vi "close references.vi"(8 "error in":errorcluster, 11 "initialized references":T1[](array[typedef])) -> (0 "error out":errorcluster)   [LabVIEW 2013]
uses:
  Controls/initialized references.ctl
  Controls/interface VI type.ctl
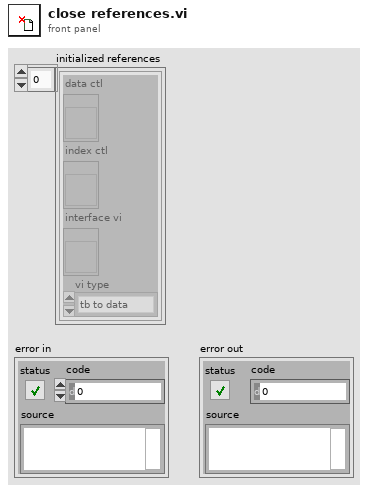
[diagram p1: front panel]
types:
  T1 = typedef "initialized references.ctl" = cluster{"data ctl":refnum<vi>, "index ctl":refnum<vi>, "interface vi":refnum<vi>, "vi type":T2}
  T2 = typedef "interface VI type.ctl" = enum16{"tb to data", "data to tb"}
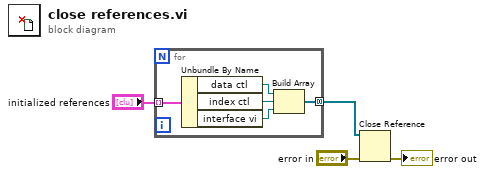
[diagram p0: block diagram]
diagram:
  n1 = for {
    tunnel: "initialized references" -> [w9] mode=indexing
    tunnel: [w5] -> w1 mode=concatenating
    n2 = Unbundle By Name(w9) -> ("data ctl"=w6:refnum<vi>, "index ctl"=w7:refnum<vi>, "interface vi"=w8:refnum<vi>)
    n3 = Build Array(w6, w7, w8) -> (w5:refnum<vi>[])
  }
  n4 = Close Reference(reference=w1, error in (no error)="error in") -> (error out=→"error out":errorcluster)
